vi "Setup DAQ.vi"(7 "buffer size multiple":dbl=2.0, 8 "error in (no error)":errorcluster, 11 "Sampling info in":T1={"Channels"=[], "Sampling freq"=0, "Output freq"=0, "Update freq"=0, "Steps per rev"=0, "Counts per rev"=0, "Amplifier"="", "Motor driver"="", "Step bit"=0, "Max speed"=0.0, "Max accel"=0.0, "Pos gain"=0.0, "Vel gain"=0.0, "counter"="Dev1/ctr0"} {"Channels"."Hi cutoff" items=["500"=500.0, "1k"=1000.0, "5k"=5000.0, "10k"=10000.0, "20k"=20000.0]; "Channels"."Lo cutoff" items=["0.1"=0.1, "1"=1.0, "10"=10.0, "100"=100.0, "300"=300.0]; "Channels"."Gain" items=["x100"=100, "x1000"=1000, "x10000"=10000]}) -> (0 "error out":errorcluster, 1 "start time":timestamp, 2 "Run info":T3, 3 "Sampling info out":T1={"Channels"=[], "Sampling freq"=0, "Output freq"=0, "Update freq"=0, "Steps per rev"=0, "Counts per rev"=0, "Amplifier"="", "Motor driver"="", "Step bit"=0, "Max speed"=0.0, "Max accel"=0.0, "Pos gain"=0.0, "Vel gain"=0.0, "counter"="Dev1/ctr0"} {"Channels"."Hi cutoff" items=["500"=500.0, "1k"=1000.0, "5k"=5000.0, "10k"=10000.0, "20k"=20000.0]; "Channels"."Lo cutoff" items=["0.1"=0.1, "1"=1.0, "10"=10.0, "100"=100.0, "300"=300.0]; "Channels"."Gain" items=["x100"=100, "x1000"=1000, "x10000"=10000]}, 4 "output delay":dbl)   [LabVIEW 2012]
uses:
  Sampling info.ctl
  Channel.ctl
  Run info.ctl
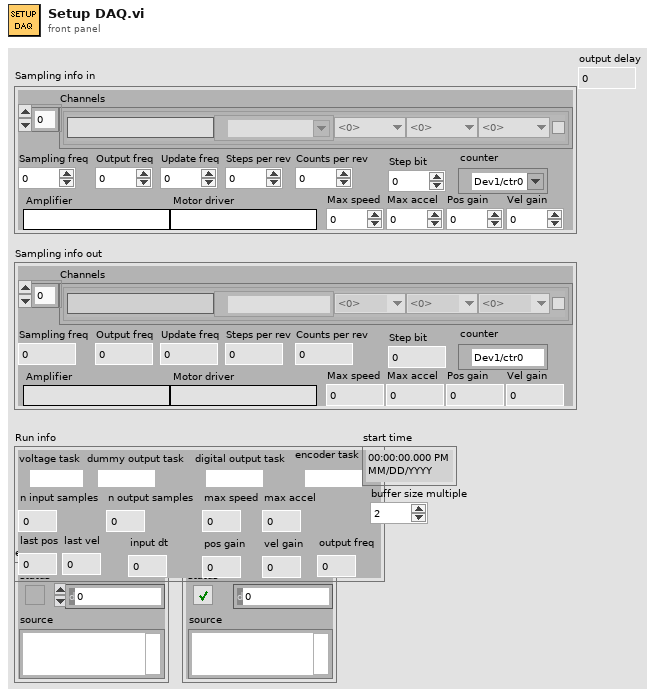
[diagram p1: front panel]
types:
  T1 = typedef "Sampling info.ctl" = cluster{"Channels":T2[], "Sampling freq":i32, "Output freq":i32, "Update freq":i32, "Steps per rev":i32, "Counts per rev":i32, "Amplifier":string, "Motor driver":string, "Step bit":u8, "Max speed":dbl, "Max accel":dbl, "Pos gain":dbl, "Vel gain":dbl, "counter":tag}
  T2 = typedef "Channel.ctl" = cluster{"Name":string, "Chan":tag, "Gain":u16, "Lo cutoff":dbl, "Hi cutoff":dbl, "Notch":bool}
  T3 = typedef "Run info.ctl" = cluster{"voltage task":refnum<k21>, "dummy output task":refnum<k21>, "digital output task":refnum<k21>, "encoder task":refnum<k21>, "n input samples":i32, "n output samples":i32, "max speed":dbl, "max accel":dbl, "last pos":dbl, "last vel":dbl, "pos gain":dbl, "vel gain":dbl, "input dt":dbl, "output freq":dbl}
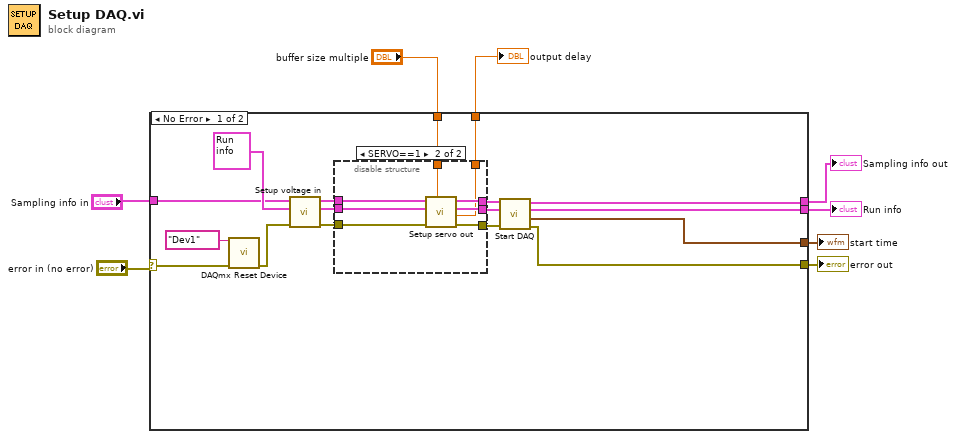
[diagram p0: block diagram]
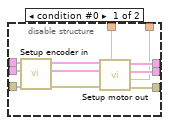
[diagram p2: hidden frame]
diagram:
  n1 = case shown="No Error" "error in (no error)" {
    selector: "error in (no error)" -> [w24 w45]
    tunnel: "Sampling info in" -> [w21 w46]
    tunnel: [w15 w45] -> w6
    tunnel: [w17 w46] -> w4
    tunnel: [w16 _] -> w5
    tunnel: [w14 _] -> w3
    tunnel: "buffer size multiple" -> [w10 _]
    tunnel: [w9 _] -> w1
    frame No Error {
      n2 = call <vilib>:"DAQmx Reset Device.vi"("device in"=tag "Dev1", "error in"=w24) -> ("error out"=w23:errorcluster)  [unwired: 13 in]
      n3 = call "Setup voltage in.vi"("error in (no error)"=w23, "Run info in"=T3 {"voltage task"="", "dummy output task"="", "digital output task"="", "encoder task"="", "n input samples"=0, "n output samples"=0, "max speed"=0.0, "max accel"=0.0, "last pos"=0.0, "last vel"=0.0, "pos gain"=0.0, "vel gain"=0.0, "input dt"=0.0, "output freq"=0.0}, "Sampling info in"=w21) -> ("error out"=w11:errorcluster, "Run info"=w12:T3, "Sampling info out"=w13:T1)  [unwired: 6 in]
      n4 = disable-structure shown="SERVO==1" {
        disable-tunnel: [w36 w41] -> w20
        disable-tunnel: [w35 w40] -> w19
        disable-tunnel: [w34 w39] -> w18
        disable-tunnel: w13 -> [w33 w44]
        disable-tunnel: w12 -> [w32 w43]
        disable-tunnel: w11 -> [w31 w42]
        disable-tunnel: w10 -> [w27 w38]
        disable-tunnel: [w26 w37] -> w9
        frame condition #0 {
          n5 = call "Setup encoder in.vi"("error in (no error)"=w31, "Run info in"=w32, "Sampling info in"=w33) -> ("error out"=w28:errorcluster, "Run info"=w29:T3, "Sampling info out"=w30:T1)  [unwired: 6 in]
          n6 = call "Setup motor out.vi"("buffer size multiple"=w27, "error in (no error)"=w28, "Run info in"=w29, "Sampling info in"=w30) -> ("error out"=w34:errorcluster, "output delay"=w26:dbl, "Run info"=w35:T3, "Sampling info out"=w36:T1)  [unwired: 4 in]
        }
        frame condition #1 (active) {
          n7 = call "Setup servo out.vi"("buffer size multiple"=w38, "error in (no error)"=w42, "Run info in"=w43, "Sampling info in"=w44) -> ("error out"=w39:errorcluster, "output delay"=w37:dbl, "Run info"=w40:T3, "Sampling info out"=w41:T1)  [unwired: 4 in]
        }
      }
      n8 = call "Start DAQ.vi"("error in (no error)"=w18, "Run info in"=w19, "Sampling info in"=w20) -> ("error out"=w15:errorcluster, "start time"=w14:timestamp, "Run info"=w16:T3, "Sampling info out"=w17:T1)  [unwired: 5 in]
    }
    frame Error {
    }
  }
  "error out" <- w6
  "Run info" <- w5
  "Sampling info out" <- w4
  "start time" <- w3
  "output delay" <- w1
